vi "Copy File.vi"(8 "error in":errorcluster, 9 "overwrite (F)":bool, 10 "target path (use dialog)":path, 11 "source path":path) -> (0 "error out":errorcluster, 3 "new path":path)   [LabVIEW 2025, in "File System.lvlib"]
uses:
  File System.lvlib
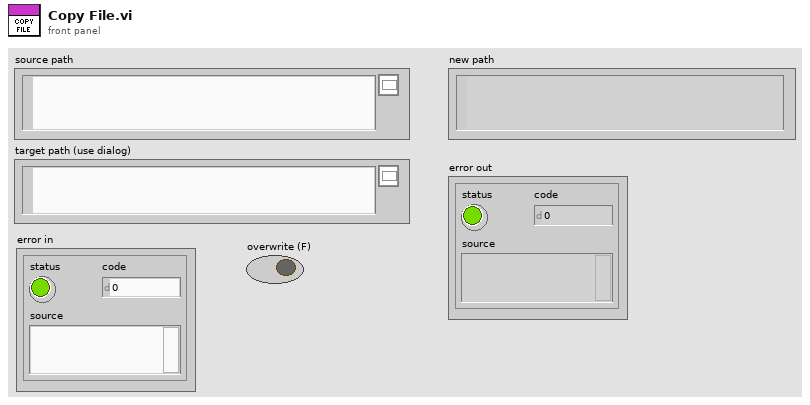
[diagram p1: front panel]
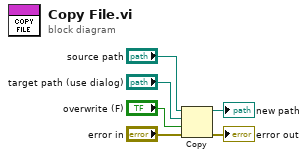
[diagram p0: block diagram]
diagram:
  n1 = Copy(8:"error in", 9:"overwrite (F)", 10:"target path (use dialog)", 11:"source path") -> (0:→"error out":errorcluster, 3:→"new path":path)  [unwired: 1 in, 1 out]
